vi "jsq_send.vi"(10 "Sequence File":path, 11 "vi path":path) -> ()   [LabVIEW 2015, in "oskar_tools.lvlib"]
uses:
  oskar_tools.lvlib
  Global.vi
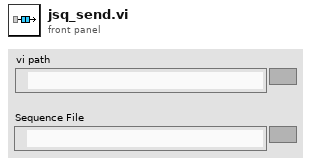
[diagram p1: front panel]
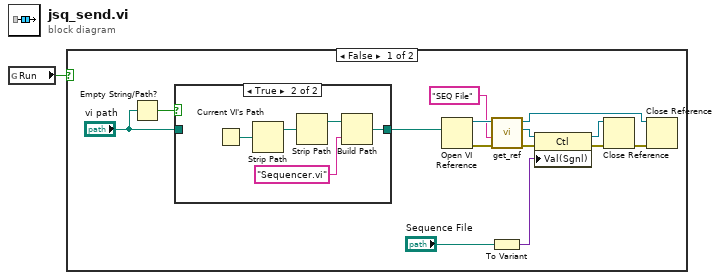
[diagram p0: block diagram]
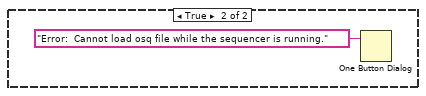
[diagram p3: hidden frame]
diagram:
  n1 = global read "Global.vi" "Run"() -> (w1:bool)
  n2 = case shown="False" w1 {
    frame False {
      n3 = Empty String/Path?(string/path="vi path") -> (empty?=w4:bool)
      n4 = case shown="True" w4 {
        tunnel: [w16 w17] -> w3
        tunnel: "vi path" -> [w16 _]
        frame False {
        }
        frame True {
          n5 = Current VI's Path() -> (path=w18:path)
          n6 = Strip Path(path=w18) -> (stripped path=w19:path)  [unwired: 1 out]
          n7 = Strip Path(path=w19) -> (stripped path=w20:path)  [unwired: 1 out]
          n8 = Build Path(base path=w20, name or relative path="Sequencer.vi") -> (appended path=w17:path)
        }
      }
      n9 = Open VI Reference(vi path=w3) -> (vi reference=w15:refnum<vi>, error out=w13:errorcluster)  [unwired: 5 in]
      n10 = call "get_ref.vi"("error in (no error)"=w13, "Name"="SEQ File", "VI reference"=w15) -> ("error out"=w9:errorcluster, "Ctrl reference out"=w6:refnum<vi>, "VI reference out"=w7:refnum<vi>)  [unwired: 5 in, 1 out]
      n11 = To Variant(anything="Sequence File") -> (Variant=w8:variant)
      n12 = property class="Ctl"(reference=w6, error in=w9, "Val(Sgnl)"=w8) -> (reference out=w11:refnum<vi>, error out=w10:errorcluster)
      n13 = Close Reference(reference=w11, error in (no error)=w10) -> (error out=w12:errorcluster)
      n14 = Close Reference(reference=w7, error in (no error)=w12) -> ()  [unwired: 1 out]
    }
    frame True {
      n15 = One Button Dialog(message="Error:  Cannot load osq file while the sequencer is running." ("error source (\" \")")) -> ()  [unwired: 1 in, 1 out]
    }
  }
